vi "FTW-JSON-Minify.vi"(1 "JSON String":string) -> (0 "Minified JSON":string)   [LabVIEW 2012]
panel:
  # "Inputs"
  # "Outputs"
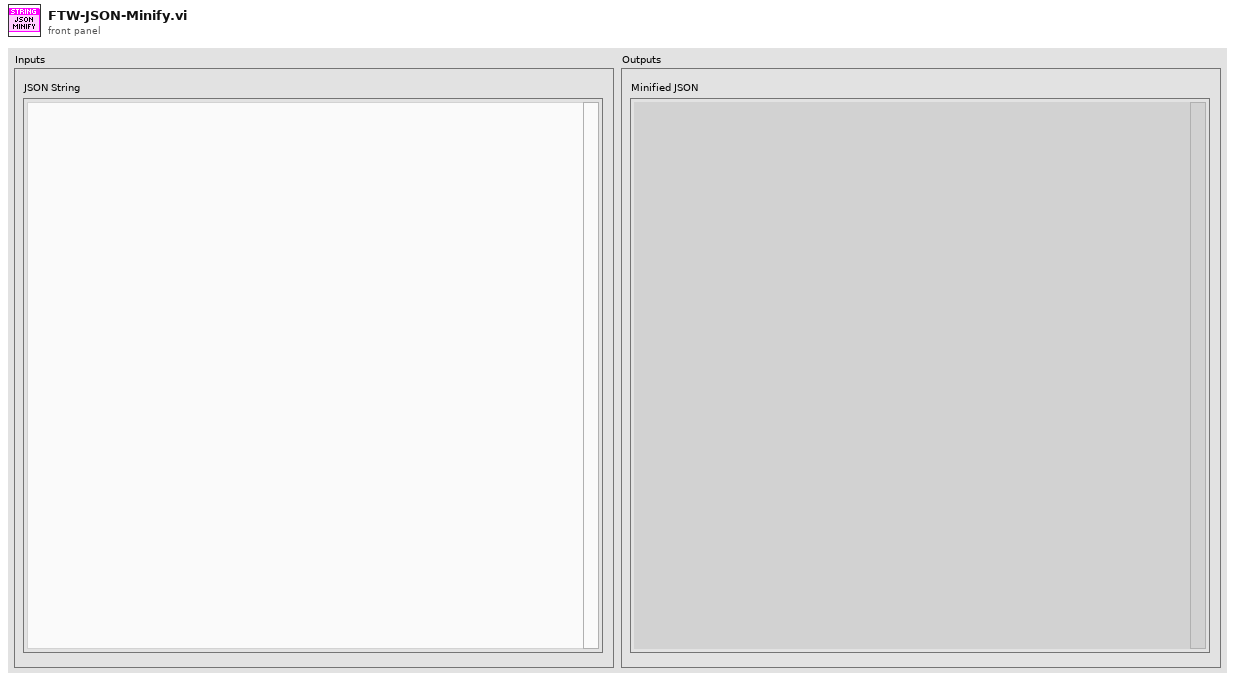
[diagram p1: front panel]
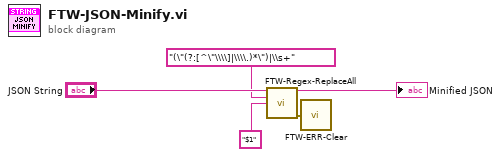
[diagram p0: block diagram]
diagram:
  n1 = call "FTW-Regex-ReplaceAll.vi"("String"="JSON String", "Search for (Regular Expression)"="(\"(?:[^\"\\\\]|\\\\.)*\")|\\s+" ("Search for"), "Replace with"="$1") -> ("String out"=→"Minified JSON":string, "error out"=w1:errorcluster)  [unwired: 10 in, 1 out]
  n2 = call "FTW-ERR-Clear.vi"("error to snuff"=w1) -> ()  [unwired: 1 out]
